vi "NI VeriStand - Get Custom Device Waveform Data.vi"(8 "error in (no error)":errorcluster, 11 "Waveform Ref in":T3 format="%.0x") -> (0 "error out":errorcluster, 1 "Waveform":T1, 2 "Waveform Name":string, 3 "Waveform Ref out":T3 format="%.0x", 4 "Found":bool, 5 "GUID":string)   [LabVIEW 2026, in "Custom Devices Storage.lvlib"]
uses:
  Custom Devices Storage.lvlib
  <vilib>/NI VeriStand/Custom Device API/Custom Device Item Ref.ctl
  <vilib>/NI VeriStand/Custom Device API/Custom Device Waveform.ctl
  <vilib>/NI VeriStand/Custom Device API/Custom Device Waveform DataType.ctl
  C:/Users/Administrator/Desktop/Jatin/All DNC DLLs/NationalInstruments.VeriStand.SystemDefinitionAPI.dll
  Jatin/All DNC DLLs/NationalInstruments.VeriStand.SystemDefinitionAPI.dll
  <vilib>/NI VeriStand/Custom Device API/Custom Device API.lvlib
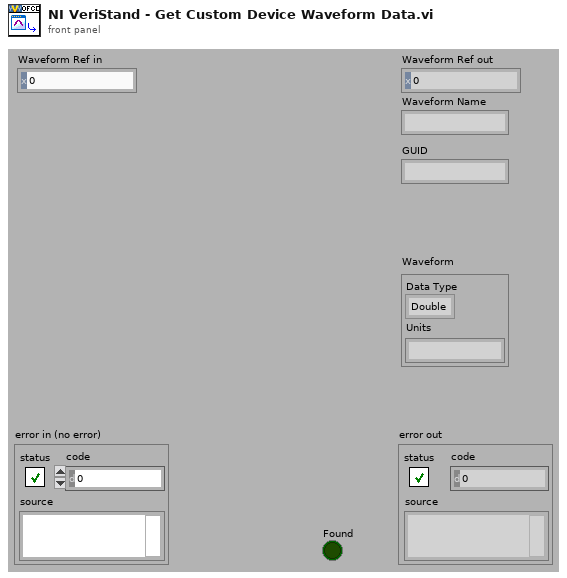
[diagram p1: front panel]
types:
  T1 = typedef "Custom Device API.lvlib/Custom Device Waveform.ctl" = cluster{"Data Type":T2, "Units":string}
  T2 = typedef "Custom Device API.lvlib/Custom Device Waveform DataType.ctl" = enum16{"Double", "Complex Double"}
  T3 = typedef "Custom Device API.lvlib/Custom Device Item Ref.ctl" = u64
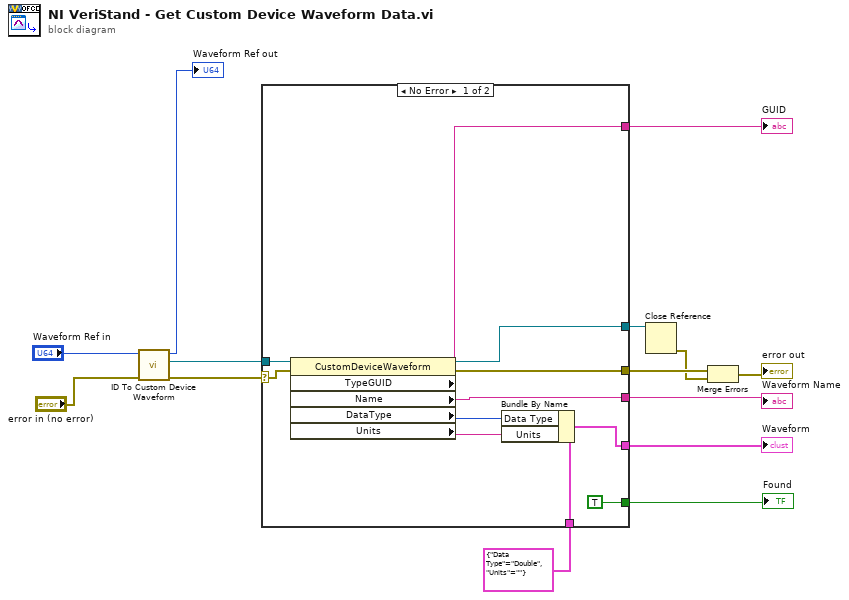
[diagram p0: block diagram]
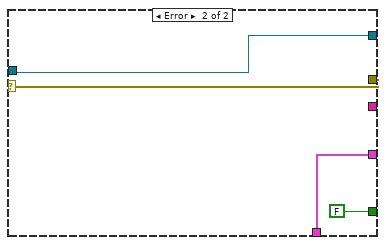
[diagram p2: hidden frame]
diagram:
  n1 = call "ID To Custom Device Waveform.vi"("error in (no error)"="error in (no error)", "ID in"="Waveform Ref in") -> ("error out"=w12:errorcluster, "NationalInstruments.VeriStand.SystemDefinitionAPI.CustomDeviceWaveform"=w11:refnum<k39>, "ID out"=→"Waveform Ref out":u64)  [unwired: 7 in]
  n2 = case shown="No Error" w12 {
    selector: w12 -> [w23 w27]
    tunnel: w11 -> [w25 w26]
    tunnel: [w24 _] -> w9
    tunnel: [w22 w27] -> w8
    tunnel: [w21 _] -> w7
    tunnel: [TRUE FALSE] -> w6
    tunnel: [w18 w28] -> w5
    tunnel: T1 {"Data Type"=enum."Double", "Units"=""} ("Waveform") -> [w19 w28]
    tunnel: [w15 w26] -> w3
    frame No Error {
      n3 = property class="CustomDeviceWaveform"(reference=w25, error in=w23) -> (reference out=w15:refnum<k39>, error out=w22:errorcluster, "TypeGUID"=w24:string, "Name"=w21:string, "DataType"=w17:i32, "Units"=w16:string)
      n4 = Bundle By Name(cluster=w19, "Data Type"=w17, "Units"=w16) -> (w18:T1)
    }
    frame Error {
    }
  }
  "Waveform" <- w5
  "Found" <- w6
  "GUID" <- w9
  "Waveform Name" <- w7
  n5 = Close Reference(reference=w3) -> (error out=w1:errorcluster)  [unwired: 1 in]
  n6 = Merge Errors(w8, w1) -> (→"error out":errorcluster)
